vi "Determine_Meas_Analysis.vi"(0 "Analogue Channels":T1[](array[typedef])=[{"Colour"=0, "Inst type"=enum."Pitot-static tube", "Inst name"="Manometer voltage", "Symbol"="U", "Code name"="", "Extra Info"="U", "Inst Array"=enum."PWA", "Index"=0, "Voltage Index"=0, "Extra Titles"=[], "Extra Values"=[]}, {"Colour"=0, "Inst type"=enum."Pitot-static tube", "Inst name"="Manometer voltage", "Symbol"="U", "Code name"="", "Extra Info"="U", "Inst Array"=enum."PWA", "Index"=0, "Voltage Index"=0, "Extra Titles"=[], "Extra Values"=[]}]) -> (1 "Analysis Info Cluster":T1[](array[typedef])=[{"Colour"=0, "Inst type"=enum."Pitot-static tube", "Inst name"="Manometer voltage", "Symbol"="U", "Code name"="", "Extra Info"="U", "Inst Array"=enum."PWA", "Index"=0, "Voltage Index"=0, "Extra Titles"=[], "Extra Values"=[]}, {"Colour"=0, "Inst type"=enum."Pitot-static tube", "Inst name"="Manometer voltage", "Symbol"="U", "Code name"="", "Extra Info"="U", "Inst Array"=enum."PWA", "Index"=0, "Voltage Index"=0, "Extra Titles"=[], "Extra Values"=[]}, {"Colour"=0, "Inst type"=enum."Pitot-static tube", "Inst name"="Manometer voltage", "Symbol"="U", "Code name"="", "Extra Info"="U", "Inst Array"=enum."PWA", "Index"=0, "Voltage Index"=0, "Extra Titles"=[], "Extra Values"=[]}, {"Colour"=0, "Inst type"=enum."Pitot-static tube", "Inst name"="Manometer voltage", "Symbol"="U", "Code name"="", "Extra Info"="U", "Inst Array"=enum."PWA", "Index"=0, "Voltage Index"=0, "Extra Titles"=[], "Extra Values"=[]}, {"Colour"=0, "Inst type"=enum."Pitot-static tube", "Inst name"="Manometer voltage", "Symbol"="U", "Code name"="", "Extra Info"="U", "Inst Array"=enum."PWA", "Index"=0, "Voltage Index"=0, "Extra Titles"=[], "Extra Values"=[]}, {"Colour"=0, "Inst type"=enum."Pitot-static tube", "Inst name"="Manometer voltage", "Symbol"="U", "Code name"="", "Extra Info"="U", "Inst Array"=enum."PWA", "Index"=0, "Voltage Index"=0, "Extra Titles"=[], "Extra Values"=[]}, {"Colour"=0, "Inst type"=enum."Pitot-static tube", "Inst name"="Manometer voltage", "Symbol"="U", "Code name"="", "Extra Info"="U", "Inst Array"=enum."PWA", "Index"=0, "Voltage Index"=0, "Extra Titles"=[], "Extra Values"=[]}, {"Colour"=0, "Inst type"=enum."Pitot-static tube", "Inst name"="Manometer voltage", "Symbol"="U", "Code name"="", "Extra Info"="U", "Inst Array"=enum."PWA", "Index"=0, "Voltage Index"=0, "Extra Titles"=[], "Extra Values"=[]}], 2 "Analysis Type Array":T4[](array[typedef])=[{"Analysis type"=enum."Slow Response", "Indicies"=[], "Name"="", "Inst Array"=enum."PWA", "Info index"=0}, {"Analysis type"=enum."Slow Response", "Indicies"=[], "Name"="", "Inst Array"=enum."PWA", "Info index"=0}, {"Analysis type"=enum."Slow Response", "Indicies"=[], "Name"="", "Inst Array"=enum."PWA", "Info index"=0}])   [LabVIEW 2010]
uses:
  Controls/Analysis_info_cluster.ctl
  Controls/Inst_type.ctl
  Controls/Instrument_Array.ctl
  Controls/Analysis_type_cluster.ctl
  Controls/Analysis_type_Enum.ctl
  Globals/Meas_global.vi
  Globals/LDA_meas_global_1.vi
  Globals/LDA_meas_global_2.vi
  Acquisition/PWA/PWAtasksGLOBAL.vi
panel:
  out "output cluster":T1={"Colour"=0, "Inst type"=enum."Pitot-static tube", "Inst name"="Manometer voltage", "Symbol"="U", "Code name"="", "Extra Info"="U", "Inst Array"=enum."PWA", "Index"=0, "Voltage Index"=0, "Extra Titles"=[], "Extra Values"=[]}
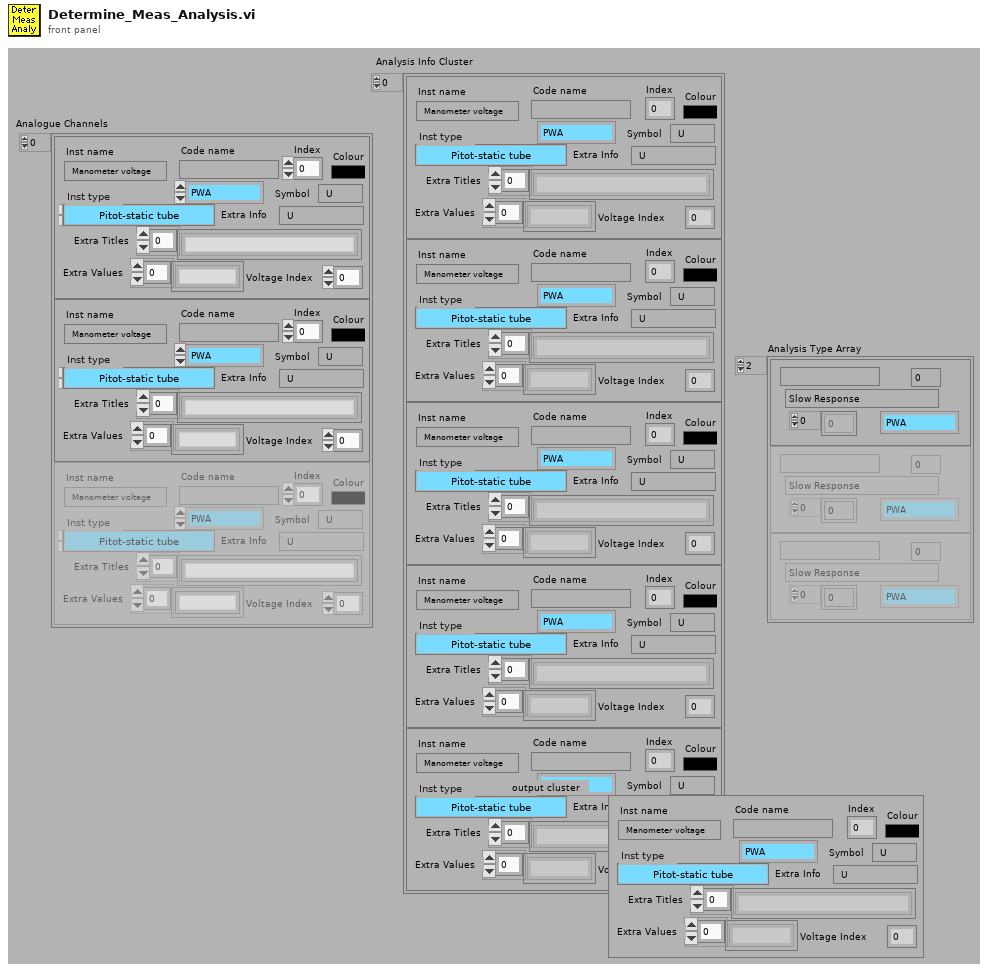
[diagram p1: front panel]
types:
  T1 = typedef "Analysis_info_cluster.ctl" = cluster{"Colour":u32, "Inst type":T2, "Inst name":string, "Symbol":string, "Code name":string, "Extra Info":string, "Inst Array":T3, "Index":i32, "Voltage Index":i32, "Extra Titles":string[], "Extra Values":string[]}
  T2 = typedef "Inst_type.ctl" = enum16{"Propeller anemometer", "Raw voltage", "Pressure Transducer", "Pitot-static tube", "Preston tube", "Hot wire", "Cross wire 1", "Cross wire 2", "Generic Linear", "Generic Polynomial", "Generic BackPoly", "Fast FID", "Thermocouple", "Cold wire", "Pulsed Wire", "LDA Vel", "LDA Tran time", "LDA Arr time"}
  T3 = typedef "Instrument_Array.ctl" = enum16{"PWA", "LDA", "Analogue"}
  T4 = typedef "Analysis_type_cluster.ctl" = cluster{"Analysis type":T5, "Indicies":i32[], "Name":string, "Inst Array":T3, "Info index":i32}
  T5 = typedef "Analysis_type_Enum.ctl" = enum16{"Slow Response", "Fast Response", "Weighted Fast Response", "Fast FID", "Weighted Fast FID", "Cross Wire", "Weighted Cross Wire", "Weighted LDA"}
  T6 = cluster{"Name":string, "X":dbl, "Y":dbl, "Z":dbl}[]
  T7 = typedef "BSA_info_Cluster.ctl" = cluster{"GPIB Address":string, "No of Check Bytes":i32, "Extra Info":string, "COLOUR":u32, "Wavelength (nm)":dbl}
  T8 = typedef "Post_Process.ctl" = enum16{"Take New Data", "Post Process Raw Data File"}
  T9 = typedef "PWA_Data.ctl" = enum16{"No PWA Data", "One Ch PWA"}
  T10 = cluster{"Name":string, "X":dbl, "Y":dbl, "Z":dbl}
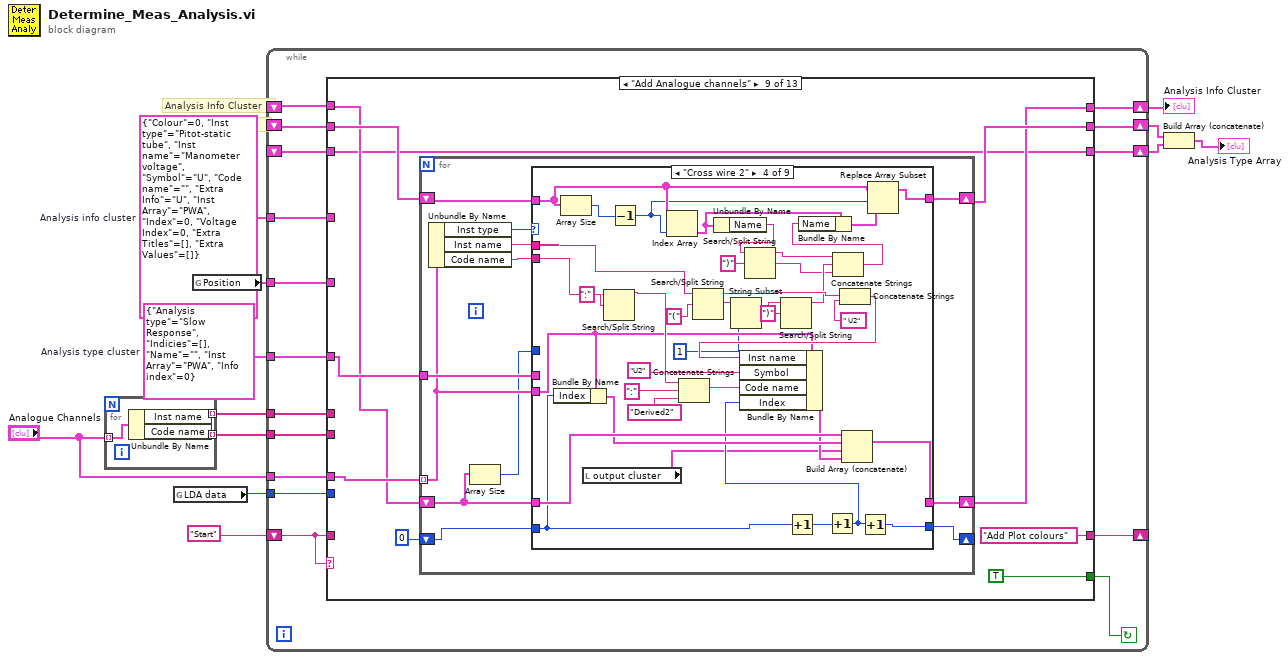
[diagram p0: block diagram]
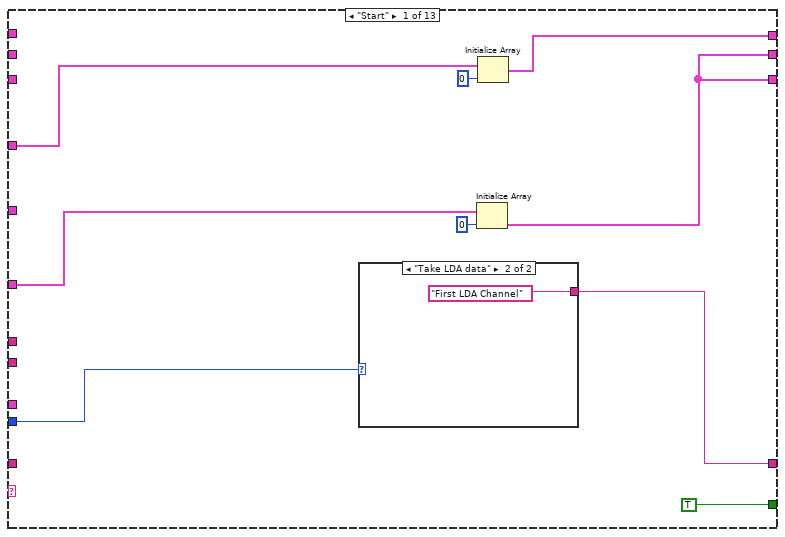
[diagram p2: hidden frame]
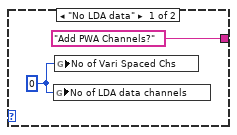
[diagram p3: hidden frame]
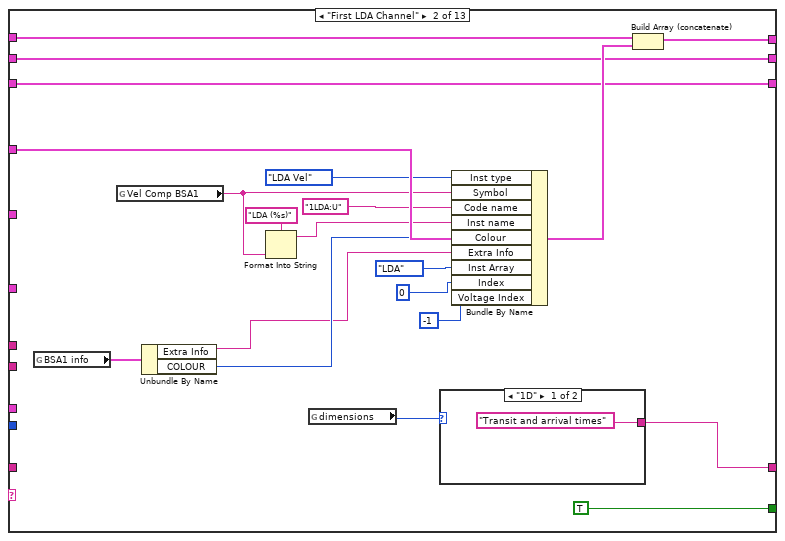
[diagram p4: hidden frame]
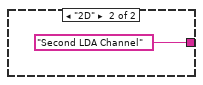
[diagram p5: hidden frame]
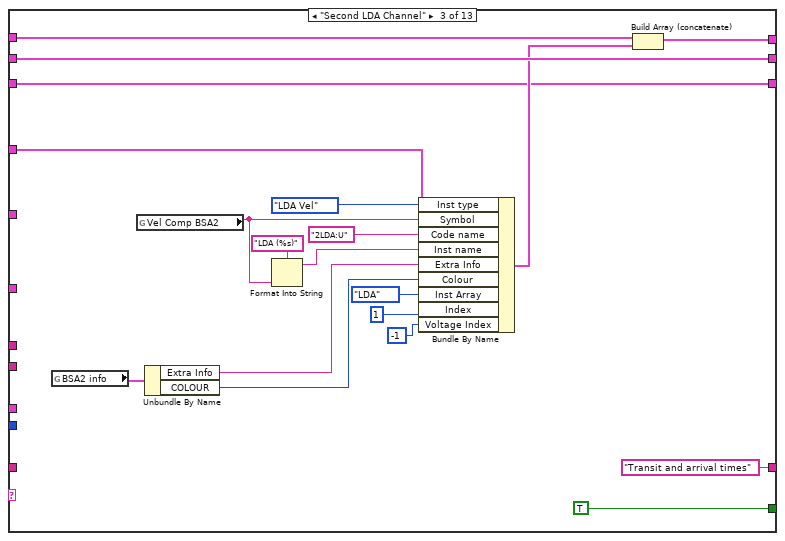
[diagram p6: hidden frame]
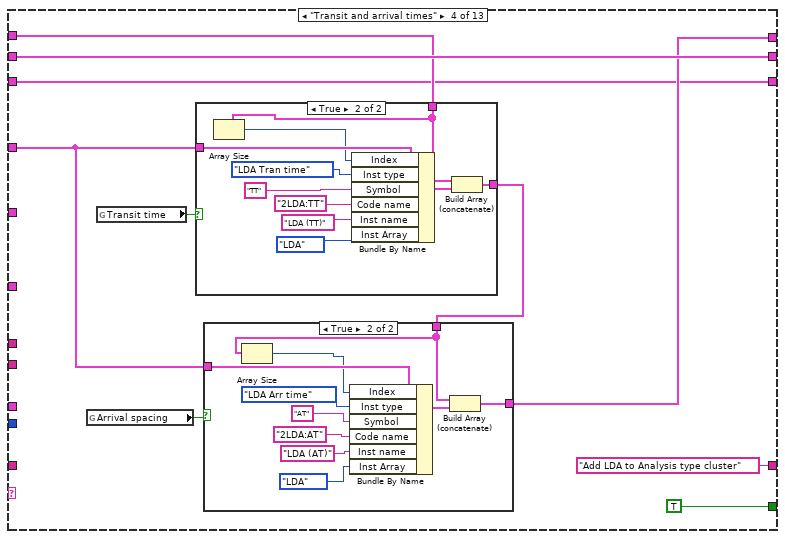
[diagram p7: hidden frame]
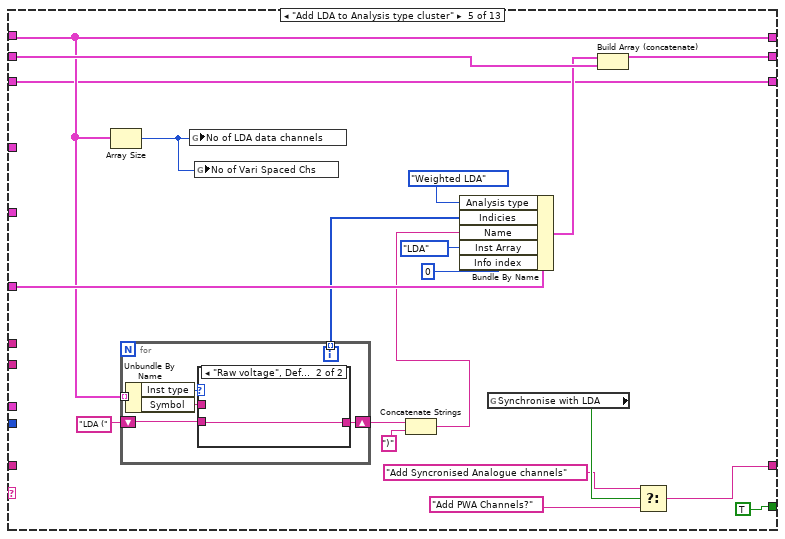
[diagram p10: hidden frame]
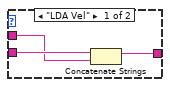
[diagram p11: hidden frame]
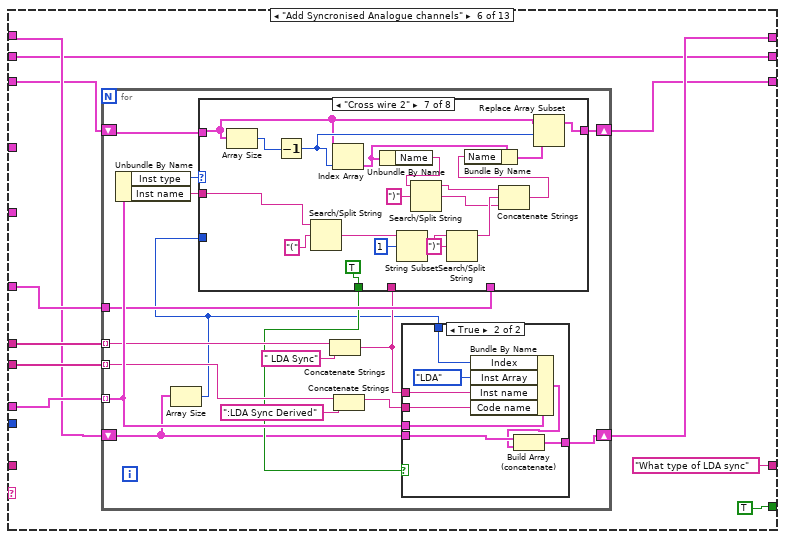
[diagram p12: hidden frame]
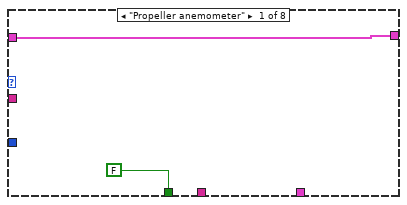
[diagram p14: hidden frame]
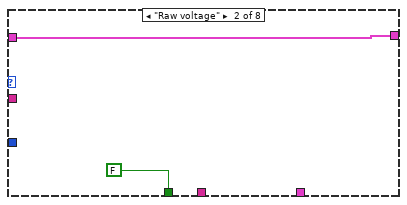
[diagram p15: hidden frame]
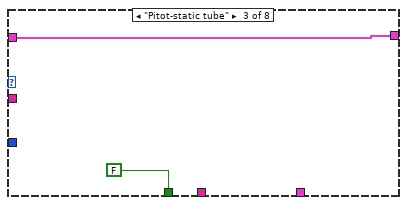
[diagram p16: hidden frame]
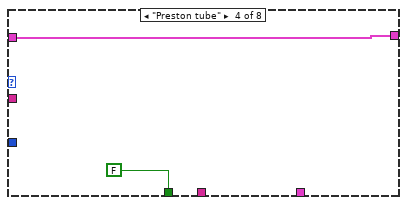
[diagram p17: hidden frame]
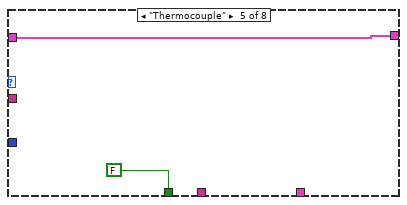
[diagram p18: hidden frame]
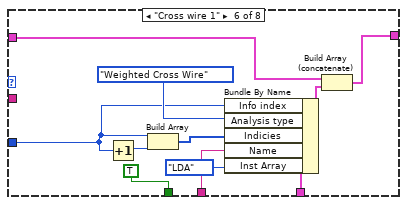
[diagram p19: hidden frame]
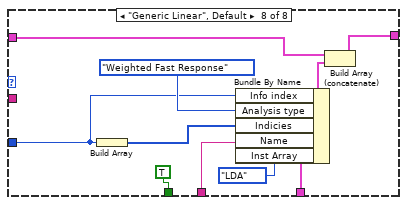
[diagram p20: hidden frame]
diagram:
  w11 = T4 {"Analysis type"=enum."Slow Response", "Indicies"=[], "Name"="", "Inst Array"=enum."PWA", "Info index"=0}  # Analysis type cluster
  w12 = T1 {"Colour"=0, "Inst type"=enum."Pitot-static tube", "Inst name"="Manometer voltage", "Symbol"="U", "Code name"="", "Extra Info"="U", "Inst Array"=enum."PWA", "Index"=0, "Voltage Index"=0, "Extra Titles"=[], "Extra Values"=[]}  # Analysis info cluster
  # "Analysis Type Array"
  # "Analysis Info Cluster"
  n1 = for {
    tunnel: "Analogue Channels" -> [w15] mode=indexing
    tunnel: [w14] -> w6 mode=indexing
    tunnel: [w13] -> w5 mode=indexing
    n2 = Unbundle By Name(w15) -> ("Inst name"=w14:string, "Code name"=w13:string)
  }
  n3 = global read "Meas_global.vi" "LDA data"() -> (w10:enum16{"No LDA data", "Take LDA data"})
  n4 = global read "Meas_global.vi" "Position"() -> (w8:T6)
  n5 = while {
    tunnel: w5 -> [w20]
    tunnel: w6 -> [w21]
    tunnel: "Analogue Channels" -> [w22]
    tunnel: w8 -> [w23]
    tunnel: w10 -> [w24]
    tunnel: w11 -> [w27]
    tunnel: w12 -> [w28]
    shift-left: _ -> [w25]
    shift-right: [w29] -> w2
    shift-left: _ -> [w26]
    shift-right: [w30] -> w9
    shift-right: [w19] -> _
    shift-left: "Start" -> [w18]
    shift-right: [w17] -> w3
    shift-left: _ -> [w16]
    stop <- w31 continue-if-true
    n6 = case shown="\"Add Analogue channels\"" w18 {
      tunnel: [TRUE TRUE TRUE TRUE TRUE TRUE TRUE TRUE TRUE TRUE TRUE FALSE FALSE] -> w31
      tunnel: [w38 w57 w82 w88 w129 w151 w236 w252 w286 w481 w510 w523 w544] -> w30
      tunnel: [w32 w56 w81 w93 w133 w147 w239 w249 w288 w480 w506 w520 w543] -> w29
      tunnel: w28 -> [w35 w62 w80 w89 _ _ _ w254 _ _ _ _ _]
      tunnel: w27 -> [w36 _ _ _ w135 w156 _ w251 w289 _ _ _ _]
      tunnel: w26 -> [_ w59 w83 w86 w129 w150 w236 w253 w283 w482 w510 w523 w544]
      tunnel: w25 -> [_ w56 w81 w93 w132 w147 w239 w250 w287 w480 w506 w520 w543]
      tunnel: w22 -> [_ _ _ _ _ w152 _ _ w284 _ _ _ _]
      tunnel: w24 -> [w34 _ _ _ _ _ _ _ _ _ _ _ _]
      tunnel: w23 -> [_ _ _ _ _ _ _ _ _ _ w509 _ _]
      tunnel: w21 -> [_ _ _ _ _ w155 _ _ _ _ _ _ _]
      tunnel: w20 -> [_ _ _ _ _ w154 _ _ _ _ _ _ _]
      tunnel: [w33 w48 "Transit and arrival times" "Add LDA to Analysis type cluster" w121 "What type of LDA sync" w234 "Add Analogue channels" "Add Plot colours" "Create Position Names" "End" "End" "End"] -> w19
      tunnel: w18 -> [_ _ _ _ _ _ _ _ _ _ _ _ w537]
      tunnel: [w32 w45 w67 w85 w117 w148 w233 w248 w282 w477 w507 w519 w535] -> w17
      tunnel: w16 -> [_ w45 w67 w85 w117 w149 w233 w248 w282 w477 w507 w519 w535]
      frame "Start" {
        n7 = case shown="\"Take LDA data\"" w34 {
          tunnel: ["Add PWA Channels?" "First LDA Channel"] -> w33
          frame "No LDA data" {
            w42 = 0 ("No of LDA data channels")
            n8 = global write "Meas_global.vi" "No of LDA data channels"(w42) -> ()
            n9 = global write "Meas_global.vi" "No of Vari Spaced Chs"(w42) -> ()
          }
          frame "Take LDA data" {
          }
        }
        n10 = Initialize Array(w36, 0 ("Dimension Size")) -> (w32:T4[])
        n11 = Initialize Array(w35, 0 ("Dimension Size")) -> (w38:T1[])
      }
      frame "First LDA Channel" {
        n12 = global read "LDA_meas_global_1.vi" "BSA1 info"() -> (w51:T7)
        n13 = global read "LDA_meas_global_1.vi" "Vel Comp BSA1"() -> (w54:string)
        n14 = Unbundle By Name(w51) -> ("Extra Info"=w49:string, "COLOUR"=w50:u32)
        n15 = Format Into String(format string="LDA (%s)" ("Format String"), w54) -> (resulting string=w52:string)  [unwired: 2 in, 1 out]
        n16 = global read "Meas_global.vi" "dimensions"() -> (w60:enum16{"1D", "2D"})
        n17 = case shown="\"1D\"" w60 {
          tunnel: ["Transit and arrival times" "Second LDA Channel"] -> w48
          frame "1D" {
          }
          frame "2D" {
          }
        }
        n18 = Bundle By Name(cluster=w62, "Inst type"=Inst_type."LDA Vel", "Symbol"=w54, "Code name"="1LDA:U" ("Bundle Element"), "Inst name"=w52, "Colour"=w50, "Extra Info"=w49, "Inst Array"=Instrument_Array."LDA" ("Instrument Array"), "Index"=0, "Voltage Index"=-1) -> (w58:T1)
        n19 = Build Array (concatenate)(w59, w58) -> (w57:T1[])
      }
      frame "Second LDA Channel" {
        n20 = global read "LDA_meas_global_2.vi" "BSA2 info"() -> (w73:T7)
        n21 = global read "LDA_meas_global_2.vi" "Vel Comp BSA2"() -> (w74:string)
        n22 = Unbundle By Name(w73) -> ("Extra Info"=w71:string, "COLOUR"=w72:u32)
        n23 = Format Into String(format string="LDA (%s)" ("Format String"), w74) -> (resulting string=w76:string)  [unwired: 2 in, 1 out]
        n24 = Bundle By Name(cluster=w80, "Inst type"=Inst_type."LDA Vel", "Symbol"=w74, "Code name"="2LDA:U" ("Bundle Element"), "Inst name"=w76, "Extra Info"=w71, "Colour"=w72, "Inst Array"=Instrument_Array."LDA" ("Instrument Array"), "Index"=1, "Voltage Index"=-1) -> (w75:T1)
        n25 = Build Array (concatenate)(w83, w75) -> (w82:T1[])
      }
      frame "Transit and arrival times" {
        n26 = global read "Meas_global.vi" "Arrival spacing"() -> (w91:bool)
        n27 = global read "Meas_global.vi" "Transit time"() -> (w92:bool)
        n28 = case shown="True" w92 {
          tunnel: w89 -> [_ w116]
          tunnel: w86 -> [w106 w109]
          tunnel: [w106 w112] -> w90
          frame False {
          }
          frame True {
            n29 = Array Size(array=w109) -> (size(s)=w107:i32)
            n30 = Bundle By Name(cluster=w116, "Index"=w107, "Inst type"=Inst_type."LDA Tran time", "Symbol"="TT", "Code name"="2LDA:TT" ("Bundle Element"), "Inst name"="LDA (TT)" ("Format String"), "Inst Array"=Instrument_Array."LDA") -> (w113:T1)
            n31 = Build Array (concatenate)(w109, w113) -> (w112:T1[])
          }
        }
        n32 = case shown="True" w91 {
          tunnel: w89 -> [_ w105]
          tunnel: w90 -> [w95 w98]
          tunnel: [w95 w101] -> w88
          frame False {
          }
          frame True {
            n33 = Array Size(array=w98) -> (size(s)=w97:i32)
            n34 = Bundle By Name(cluster=w105, "Index"=w97, "Inst type"=Inst_type."LDA Arr time", "Symbol"="AT", "Code name"="2LDA:AT" ("Bundle Element"), "Inst name"="LDA (AT)" ("Format String"), "Inst Array"=Instrument_Array."LDA") -> (w102:T1)
            n35 = Build Array (concatenate)(w98, w102) -> (w101:T1[])
          }
        }
      }
      frame "Add LDA to Analysis type cluster" {
        n36 = Array Size(array=w129) -> (size(s)=w123:i32)
        n37 = for {
          tunnel: w129 -> [w142] mode=indexing
          shift-right: [w138] -> w127
          shift-left: "LDA (" -> [w140]
          tunnel: [w137] -> w124 mode=indexing
          i -> [w137]
          n38 = Unbundle By Name(w142) -> ("Inst type"=w141:T2, "Symbol"=w139:string)
          n39 = case shown="\"Raw voltage\", Default" w141 {
            tunnel: w140 -> [w145 w146]
            tunnel: w139 -> [w144 _]
            tunnel: [w143 w146] -> w138
            frame "LDA Vel" {
              n40 = Concatenate Strings(w145, w144) -> (w143:string)
            }
            frame "Raw voltage", Default {
            }
          }
        }
        n41 = global write "Meas_global.vi" "No of LDA data channels"(w123) -> ()
        n42 = global write "Meas_global.vi" "No of Vari Spaced Chs"(w123) -> ()
        n43 = Concatenate Strings(w127, ")" ("Substring")) -> (w125:string)
        n44 = Bundle By Name(cluster=w135, "Analysis type"=Analysis_type_Enum."Weighted LDA", "Indicies"=w124, "Name"=w125, "Inst Array"=Instrument_Array."LDA", "Info index"=0) -> (w130:T4)
        n45 = global read "Meas_global.vi" "Synchronise with LDA"() -> (w131:bool)
        n46 = Build Array (concatenate)(w130, w132) -> (w133:T4[])
        n47 = Select(t="Add Syncronised Analogue channels", s=w131, f="Add PWA Channels?") -> (s? t:f=w121:string)
      }
      frame "Add Syncronised Analogue channels" {
        n48 = for {
          tunnel: w152 -> [w172] mode=indexing
          shift-right: [w169] -> w148
          shift-left: w149 -> [w171]
          tunnel: w156 -> [w170]
          tunnel: w155 -> [w167] mode=indexing
          tunnel: w154 -> [w166] mode=indexing
          shift-right: [w162] -> w151
          shift-left: w150 -> [w160]
          n49 = Unbundle By Name(w172) -> ("Inst type"=w173:T2, "Inst name"=w158:string)
          n50 = Array Size(array=w160) -> (size(s)=w159:i32)
          n51 = Concatenate Strings(w167, " LDA Sync" ("Substring")) -> (w168:string)
          n52 = case shown="\"Cross wire 2\"" w173 {
            tunnel: w171 -> [w183 w185 w187 w189 w191 w203 w207 w232]
            tunnel: [w183 w185 w187 w189 w191 w202 w206 w231] -> w169
            tunnel: w170 -> [_ _ _ _ _ w201 _ w230]
            tunnel: w159 -> [_ _ _ _ _ w193 _ w223]
            tunnel: w168 -> [_ _ _ _ _ w196 _ w226]
            tunnel: [FALSE FALSE FALSE FALSE FALSE TRUE TRUE TRUE] -> w161
            tunnel: w158 -> [_ _ _ _ _ _ w208 _]
            frame "Propeller anemometer" {
            }
            frame "Raw voltage" {
            }
            frame "Pitot-static tube" {
            }
            frame "Preston tube" {
            }
            frame "Thermocouple" {
            }
            frame "Cross wire 1" {
              n53 = Increment(x=w193) -> (x+1=w198:i32)
              n54 = Build Array(w193, w198) -> (w199:i32[])
              n55 = Bundle By Name(cluster=w201, "Info index"=w193, "Analysis type"=Analysis_type_Enum."Weighted Cross Wire", "Indicies"=w199, "Name"=w196, "Inst Array"=Instrument_Array."LDA") -> (w197:T4)
              n56 = Build Array (concatenate)(w203, w197) -> (w202:T4[])
            }
            frame "Cross wire 2" {
              n57 = Array Size(array=w207) -> (size(s)=w219:i32)
              n58 = Decrement(x=w219) -> (x-1=w218:i32)
              n59 = Search/Split String(string=w208, search string/char (-)="(") -> (match + rest of string=w210:string)  [unwired: 3 out]
              n60 = Index Array(array=w207, index=w218) -> (element=w216:T4)
              n61 = Unbundle By Name(w216) -> ("Name"=w215:string)
              n62 = String Subset(string=w210, offset (0)=1) -> (substring=w209:string)  [unwired: 1 out]
              n63 = Search/Split String(string=w215, search string/char (-)=")") -> (substring before match=w214:string, match + rest of string=w204:string)  [unwired: 2 out]
              n64 = Search/Split String(string=w209, search string/char (-)=")") -> (substring before match=w213:string)  [unwired: 3 out]
              n65 = Concatenate Strings(w214, w213, w204) -> (w211:string)
              n66 = Bundle By Name(cluster=w216, "Name"=w211) -> (w217:T4)
              n67 = Replace Array Subset(array=w207, new element=w217, index=w218) -> (w206:T4[])
            }
            frame "Generic Linear", Default {
              n68 = Build Array(w223) -> (w227:i32[])
              n69 = Bundle By Name(cluster=w230, "Info index"=w223, "Analysis type"=Analysis_type_Enum."Weighted Fast Response", "Indicies"=w227, "Name"=w226, "Inst Array"=Instrument_Array."LDA") -> (w229:T4)
              n70 = Build Array (concatenate)(w232, w229) -> (w231:T4[])
            }
          }
          n71 = Concatenate Strings(w166, ":LDA Sync Derived" ("Substring")) -> (w163:string)
          n72 = case shown="True" w161 {
            tunnel: w172 -> [_ w182]
            tunnel: w168 -> [_ w181]
            tunnel: w159 -> [_ w180]
            tunnel: w163 -> [_ w179]
            tunnel: [w174 w177] -> w162
            tunnel: w160 -> [w174 w176]
            frame False {
            }
            frame True {
              n73 = Bundle By Name(cluster=w182, "Index"=w180, "Inst Array"=Instrument_Array."LDA", "Inst name"=w181, "Code name"=w179) -> (w175:T1)
              n74 = Build Array (concatenate)(w176, w175) -> (w177:T1[])
            }
          }
        }
      }
      frame "What type of LDA sync" {
        n75 = global read "Meas_global.vi" "Post Process"() -> (w238:T8)
        n76 = Array Size(array=w236) -> (size(s)=w237:i32)
        n77 = case shown="\"Take New Data\"" w238 {
          tunnel: [w241 w243] -> w234
          tunnel: "Add PWA Channels?" -> [w241 w244]
          frame "Take New Data" {
          }
          frame "Post Process Raw Data File" {
            w246 = 3083254242.0  # 13/9/01 When new synchronisation routine was implemented
            n78 = global read "Meas_global.vi" "Time Data was Aquired"() -> (w247:dbl)
            n79 = Greater?(x=w247, y=w246) -> (0:w245:bool)
            n80 = Select(t=w244, s=w245, f="Add Plot colours") -> (s? t:f=w243:string)
          }
        }
        n81 = global write "Meas_global.vi" "No of Vari Spaced Chs"(w237) -> ()
      }
      frame "Add PWA Channels?" {
        n82 = global read "Meas_global.vi" "PWA Data"() -> (w256:T9)
        n83 = case shown="\"One Ch PWA\"" w256 {
          tunnel: w254 -> [_ w280]
          tunnel: w253 -> [w259 w262]
          tunnel: [w259 w278] -> w252
          tunnel: w250 -> [w258 w277]
          tunnel: w251 -> [_ w275]
          tunnel: [w258 w274] -> w249
          frame "No PWA Data" {
          }
          frame "One Ch PWA" {
            n84 = global read "PWAtasksGLOBAL.vi" "PWA Symbol"() -> (w265:string)
            n85 = Format Into String(format string="PWA (%s)", w265) -> (resulting string=w266:string)  [unwired: 2 in, 1 out]
            n86 = Array Size(array=w262) -> (size(s)=w261:i32)
            n87 = Build Array(0 ("size(s)")) -> (w270:i32[])
            n88 = Bundle By Name(cluster=w280, "Inst type"=Inst_type."Pulsed Wire", "Inst name"=w266, "Symbol"=w265, "Code name"="1PWA", "Inst Array"=Instrument_Array."PWA", "Index"=0, "Voltage Index"=-1) -> (w279:T1)
            n89 = Bundle By Name(cluster=w275, "Analysis type"=Analysis_type_Enum."Fast Response", "Indicies"=w270, "Name"=w266, "Inst Array"=Instrument_Array."PWA", "Info index"=w261) -> (w276:T4)
            n90 = Build Array (concatenate)(w277, w276) -> (w274:T4[])
            n91 = Build Array (concatenate)(w262, w279) -> (w278:T1[])
          }
        }
      }
      frame "Add Analogue channels" {
        n92 = for {
          tunnel: w284 -> [w298] mode=indexing
          shift-right: [w299] -> w288
          shift-left: w287 -> [w301]
          tunnel: w289 -> [w300]
          shift-right: [w297] -> w286
          shift-left: w283 -> [w292]
          shift-right: [w294] -> _
          shift-left: 0 -> [w295]
          n93 = Unbundle By Name(w298) -> ("Inst type"=w302:T2, "Inst name"=w293:string, "Code name"=w296:string)
          n94 = Array Size(array=w292) -> (size(s)=w291:i32)
          n95 = case shown="\"Cross wire 2\"" w302 {
            tunnel: w301 -> [w317 w332 w363 w378 w416 w431 w446 w461 w476]
            tunnel: [w316 w331 w362 w374 w415 w430 w445 w460 w475] -> w299
            tunnel: w300 -> [w315 w330 w358 _ w414 w429 w444 w459 w474]
            tunnel: w293 -> [w311 w326 w347 w393 w410 w426 w440 w455 w470]
            tunnel: w292 -> [w307 w321 w344 w390 w406 w421 w433 w447 w466]
            tunnel: w298 -> [w305 w319 w337 w389 w407 w417 w435 w450 w463]
            tunnel: [w306 w322 w346 w392 w404 w418 w434 w449 w465] -> w297
            tunnel: w296 -> [_ _ w345 w391 _ _ _ _ _]
            tunnel: w295 -> [w303 w318 w335 w384 w402 w420 w436 w451 w462]
            tunnel: [w304 w320 w334 w385 w403 w419 w432 w448 w464] -> w294
            tunnel: w291 -> [w309 w324 w342 _ w408 w423 w438 w453 w468]
            frame "Propeller anemometer" {
              n96 = Build Array(w303) -> (w312:i32[])
              n97 = Bundle By Name(cluster=w305, "Index"=w303) -> (w308:T1)
              n98 = Bundle By Name(cluster=w315, "Analysis type"=Analysis_type_Enum."Slow Response", "Indicies"=w312, "Name"=w311, "Inst Array"=Instrument_Array."Analogue", "Info index"=w309) -> (w314:T4)
              n99 = Increment(x=w303) -> (x+1=w304:i32)
              n100 = Build Array (concatenate)(w317, w314) -> (w316:T4[])
              n101 = Build Array (concatenate)(w307, w308) -> (w306:T1[])
            }
            frame "Pitot-static tube" {
              n102 = Build Array(w318) -> (w327:i32[])
              n103 = Bundle By Name(cluster=w319, "Index"=w318) -> (w323:T1)
              n104 = Bundle By Name(cluster=w330, "Analysis type"=Analysis_type_Enum."Slow Response", "Indicies"=w327, "Name"=w326, "Inst Array"=Instrument_Array."Analogue", "Info index"=w324) -> (w329:T4)
              n105 = Increment(x=w318) -> (x+1=w320:i32)
              n106 = Build Array (concatenate)(w332, w329) -> (w331:T4[])
              n107 = Build Array (concatenate)(w321, w323) -> (w322:T1[])
            }
            frame "Cross wire 1" {
              n108 = Bundle By Name(cluster=w337, "Index"=w335) -> (w336:T1)
              n109 = Increment(x=w335) -> (x+1=w341:i32)
              n110 = Increment(x=w341) -> (x+1=w340:i32)
              n111 = Search/Split String(string=w345, search string/char (-)=":" ("search char (-)")) -> (substring before match=w351:string)  [unwired: 3 out]
              n112 = Increment(x=w340) -> (x+1=w339:i32)
              n113 = Build Array(w335, w341, w340, w339) -> (w360:i32[])
              n114 = Concatenate Strings(w351, ":" ("search char (-)"), "Derived1") -> (w352:string)
              n115 = Build Array (concatenate)(w344, w336) -> (w346:T1[])
              n116 = Bundle By Name(cluster=w358, "Analysis type"=Analysis_type_Enum."Cross Wire", "Indicies"=w360, "Name"=w347, "Inst Array"=Instrument_Array."Analogue", "Info index"=w342) -> (w359:T4)
              n117 = Search/Split String(string=w347, search string/char (-)="(") -> (substring before match=w356:string)  [unwired: 3 out]
              n118 = Increment(x=w335) -> (x+1=w334:i32)
              n119 = Concatenate Strings(w356, " U1") -> (w355:string)
              n120 = Increment(x=w334) -> (x+1=w333:i32)
              n121 = Bundle By Name(cluster=w337, "Inst name"=w355, "Symbol"="U1", "Code name"=w352, "Index"=w333) -> (→"output cluster":T1)
              n122 = Build Array (concatenate)(w363, w359) -> (w362:T4[])
            }
            frame "Cross wire 2" {
              n123 = Bundle By Name(cluster=w389, "Index"=w384) -> (w388:T1)
              n124 = Array Size(array=w378) -> (size(s)=w379:i32)
              n125 = local read "output cluster"() -> (w382:T1)
              n126 = Search/Split String(string=w391, search string/char (-)=":" ("search char (-)")) -> (substring before match=w397:string)  [unwired: 3 out]
              n127 = Decrement(x=w379) -> (x-1=w377:i32)
              n128 = Index Array(array=w378, index=w377) -> (element=w375:T4)
              n129 = Concatenate Strings(w397, ":" ("search char (-)"), "Derived2") -> (w398:string)
              n130 = Search/Split String(string=w393, search string/char (-)="(") -> (substring before match=w373:string, match + rest of string=w366:string)  [unwired: 2 out]
              n131 = Unbundle By Name(w375) -> ("Name"=w372:string)
              n132 = String Subset(string=w366, offset (0)=1) -> (substring=w365:string)  [unwired: 1 out]
              n133 = Search/Split String(string=w372, search string/char (-)=")") -> (substring before match=w371:string, match + rest of string=w364:string)  [unwired: 2 out]
              n134 = Search/Split String(string=w365, search string/char (-)=")") -> (substring before match=w370:string)  [unwired: 3 out]
              n135 = Increment(x=w384) -> (x+1=w386:i32)
              n136 = Increment(x=w386) -> (x+1=w383:i32)
              n137 = Concatenate Strings(w371, w370, w364) -> (w368:string)
              n138 = Bundle By Name(cluster=w375, "Name"=w368) -> (w376:T4)
              n139 = Concatenate Strings(w373, " U2") -> (w401:string)
              n140 = Bundle By Name(cluster=w389, "Inst name"=w401, "Symbol"="U2", "Code name"=w398, "Index"=w383) -> (w387:T1)
              n141 = Build Array (concatenate)(w390, w388, w382, w387) -> (w392:T1[])
              n142 = Increment(x=w383) -> (x+1=w385:i32)
              n143 = Replace Array Subset(array=w378, new element=w376, index=w377) -> (w374:T4[])
            }
            frame "Generic Linear", Default {
              n144 = Build Array(w402) -> (w411:i32[])
              n145 = Bundle By Name(cluster=w414, "Analysis type"=Analysis_type_Enum."Fast Response", "Indicies"=w411, "Name"=w410, "Inst Array"=Instrument_Array."Analogue", "Info index"=w408) -> (w413:T4)
              n146 = Bundle By Name(cluster=w407, "Index"=w402) -> (w405:T1)
              n147 = Increment(x=w402) -> (x+1=w403:i32)
              n148 = Build Array (concatenate)(w416, w413) -> (w415:T4[])
              n149 = Build Array (concatenate)(w406, w405) -> (w404:T1[])
            }
            frame "Raw voltage" {
              n150 = Build Array(w420) -> (w427:i32[])
              n151 = Bundle By Name(cluster=w417, "Index"=w420) -> (w422:T1)
              n152 = Increment(x=w420) -> (x+1=w419:i32)
              n153 = Bundle By Name(cluster=w429, "Analysis type"=Analysis_type_Enum."Slow Response", "Indicies"=w427, "Name"=w426, "Inst Array"=Instrument_Array."Analogue", "Info index"=w423) -> (w428:T4)
              n154 = Build Array (concatenate)(w421, w422) -> (w418:T1[])
              n155 = Build Array (concatenate)(w431, w428) -> (w430:T4[])
            }
            frame "Fast FID" {
              n156 = Build Array(w436) -> (w441:i32[])
              n157 = Bundle By Name(cluster=w435, "Index"=w436) -> (w437:T1)
              n158 = Increment(x=w436) -> (x+1=w432:i32)
              n159 = Bundle By Name(cluster=w444, "Analysis type"=Analysis_type_Enum."Fast FID", "Indicies"=w441, "Name"=w440, "Inst Array"=Instrument_Array."Analogue", "Info index"=w438) -> (w443:T4)
              n160 = Build Array (concatenate)(w433, w437) -> (w434:T1[])
              n161 = Build Array (concatenate)(w446, w443) -> (w445:T4[])
            }
            frame "Preston tube" {
              n162 = Build Array(w451) -> (w456:i32[])
              n163 = Bundle By Name(cluster=w450, "Index"=w451) -> (w452:T1)
              n164 = Increment(x=w451) -> (x+1=w448:i32)
              n165 = Bundle By Name(cluster=w459, "Analysis type"=Analysis_type_Enum."Slow Response", "Indicies"=w456, "Name"=w455, "Inst Array"=Instrument_Array."Analogue", "Info index"=w453) -> (w458:T4)
              n166 = Build Array (concatenate)(w447, w452) -> (w449:T1[])
              n167 = Build Array (concatenate)(w461, w458) -> (w460:T4[])
            }
            frame "Thermocouple" {
              n168 = Build Array(w462) -> (w471:i32[])
              n169 = Bundle By Name(cluster=w463, "Index"=w462) -> (w467:T1)
              n170 = Bundle By Name(cluster=w474, "Analysis type"=Analysis_type_Enum."Slow Response", "Indicies"=w471, "Name"=w470, "Inst Array"=Instrument_Array."Analogue", "Info index"=w468) -> (w473:T4)
              n171 = Increment(x=w462) -> (x+1=w464:i32)
              n172 = Build Array (concatenate)(w466, w467) -> (w465:T1[])
              n173 = Build Array (concatenate)(w476, w473) -> (w475:T4[])
            }
          }
        }
      }
      frame "Add Plot colours" {
        n174 = for {
          tunnel: [w485] -> w481 mode=indexing
          tunnel: w482 -> [w483] mode=indexing
          n175 = Unbundle By Name(w483) -> ("Inst type"=w487:T2, "Colour"=w484:u32)
          n176 = case shown="\"Pulsed Wire\"" w487 {
            tunnel: [u32 13421772 u32 13421772 u32 11711154 u32 6710784 u32 13311 u32 16724736 u32 13382400 u32 10040217 u32 16711935 u32 16711935 u32 16711935 u32 65535 u32 16776960 u32 10027263 u32 10027263 w503 u32 65280 u32 65280] -> w486
            tunnel: w484 -> [_ _ _ _ _ _ _ _ _ _ _ _ _ _ _ w503 _ _]
            frame "Propeller anemometer" {
            }
            frame "Pressure Transducer" {
            }
            frame "Raw voltage" {
            }
            frame "Pitot-static tube" {
            }
            frame "Preston tube" {
            }
            frame "Hot wire" {
            }
            frame "Cross wire 1" {
            }
            frame "Cross wire 2" {
            }
            frame "Generic Linear" {
            }
            frame "Generic Polynomial" {
            }
            frame "Generic BackPoly" {
            }
            frame "Fast FID" {
            }
            frame "Thermocouple" {
            }
            frame "Cold wire" {
            }
            frame "Pulsed Wire" {
            }
            frame "LDA Vel" {
            }
            frame "LDA Tran time" {
            }
            frame "LDA Arr time" {
            }
          }
          n177 = Bundle By Name(cluster=w483, "Colour"=w486) -> (w485:T1)
        }
      }
      frame "Create Position Names" {
        n178 = for {
          tunnel: [w518] -> w511 mode=indexing
          tunnel: w506 -> [w514] mode=indexing
          tunnel: w509 -> [w516]
          i -> [w517]
          n179 = Unbundle By Name(w514) -> ("Name"=w513:string)
          n180 = Index Array(array=w516, index=w517) -> (element=w515:T10)
          n181 = Bundle By Name(cluster=w515, "Name"=w513) -> (w518:T10)
        }
        n182 = global write "Meas_global.vi" "Position"(w511) -> ()
      }
      frame "End" {
        n183 = for {
          tunnel: w523 -> [w529] mode=indexing
          shift-right: [w526] -> w521
          shift-left: 0 -> [w527]
          n184 = Unbundle By Name(w529) -> ("Inst Array"=w528:T3)
          n185 = case shown="\"Analogue\"" w528 {
            tunnel: w527 -> [w530 w533 w534]
            tunnel: [w531 w532 w534] -> w526
            frame "PWA" {
              n186 = Increment(x=w530) -> (x+1=w531:i32)
            }
            frame "LDA" {
              n187 = Increment(x=w533) -> (x+1=w532:i32)
            }
            frame "Analogue" {
            }
          }
        }
        n188 = global write "Meas_global.vi" "No of Non Analogue Chs"(w521) -> ()
      }
      frame "No Match", Default {
        n189 = Current VI's Path() -> (path=w538:path)
        n190 = Format Into String(format string="The Case\"%s\" was not Matched\nin VI named\n'%s\"" ("Format String"), w537, w538) -> (resulting string=w541:string)  [unwired: 2 in, 1 out]
        n191 = One Button Dialog(message=w541, button name ("OK")="STOP") -> (true=w539:bool)
        n192 = Stop(stop? (T)=w539) -> ()
      }
    }
  }
  "Analysis Info Cluster" <- w9
  n193 = Build Array (concatenate)(w2, w3) -> (→"Analysis Type Array":T4[])
